vi "Pre-Dig Template.vi"(6 "Call and Forget?":bool, 8 "Error In":errorcluster, 10 "Selection List In":refnum<vi>[](array[refnum]), 11 "VI In":refnum<vi>) -> (0 "Error Out":errorcluster, 2 "Selection List Out":refnum<vi>[](array[refnum]), 3 "VI Out":refnum<vi>)   [LabVIEW 2018, in "Toolkit.lvlib"]
uses:
  Toolkit.lvlib
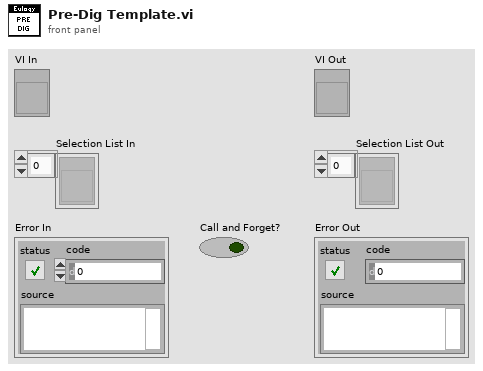
[diagram p1: front panel]
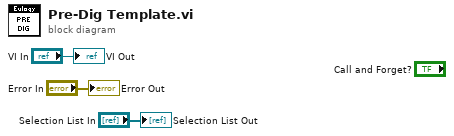
[diagram p0: block diagram]
diagram:
  "Error Out" <- "Error In"
  "Selection List Out" <- "Selection List In"
  "VI Out" <- "VI In"
